vi "Configure Analog Output Scaling.vi"(8 "error in (no error)":errorcluster, 9 "Scaling (5: 5)":i32(ring)=5 items=["3"=3, "5"=5, "10"=10], 10 "Analog Channel (0: Voltage)":i32(ring) items=["Voltage", "Current"], 11 "VISA resource name":refnum<visa-resource-name>) -> (0 "error out":errorcluster, 3 "VISA resource name out":refnum<visa-resource-name>)   [LabVIEW 2018, in "XP Power PLS600.lvlib"]
doc: "Sets the scaling level of the specified analog channel (voltage or current)."
uses:
  XP Power PLS600.lvlib
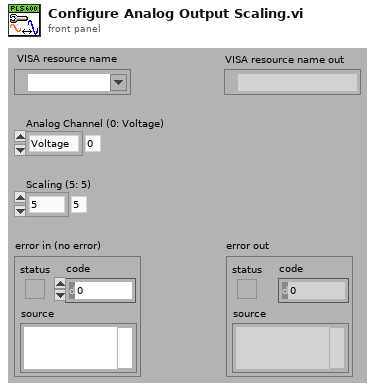
[diagram p1: front panel]
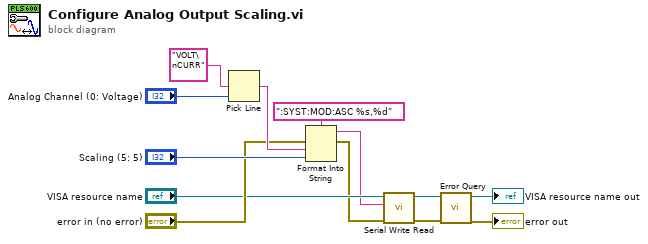
[diagram p0: block diagram]
diagram:
  n1 = Pick Line(multi-line string="VOLT\nCURR", line index="Analog Channel (0: Voltage)") -> (output string=w10:string)  [unwired: 1 in]
  n2 = Format Into String(format string=":SYST:MOD:ASC %s,%d", error in="error in (no error)", w10, "Scaling (5: 5)") -> (resulting string=w3:string, error out=w4:errorcluster)  [unwired: 1 in]
  n3 = call "Serial Write Read.vi"("error in (no error)"=w4, "Write Buffer"=w3, "VISA resource name"="VISA resource name") -> ("error out"=w1:errorcluster, "VISA resource name out"=w2:refnum<visa-resource-name>)  [unwired: 6 in, 1 out]
  n4 = call "Error Query.vi"("error in (no error)"=w1, "VISA resource name"=w2) -> ("error out"=→"error out":errorcluster, "VISA resource name out"=→"VISA resource name out":refnum<visa-resource-name>)  [unwired: 6 in, 2 out]
